vi "ARMS - LOCK.vi"(8 "error in (no error)":errorcluster, 9 "STATE":enum16{"LOCK", "UNLOCK"}(ring), 11 "SIDE":enum16{"LEFT", "RIGHT"}(ring)) -> (0 "error out":errorcluster, 3 "GET value":bool, 4 "previous GET\nvalue":bool)   [LabVIEW 2023]
uses:
  Global INIT.vi
  <vilib>/Rock Robotics/WPI/Solenoid/WPI_SolenoidValue.ctl
  <vilib>/Rock Robotics/WPI/Solenoid/WPI_SolenoidSetEnum.vi
  Global stack names.vi
  <vilib>/Rock Robotics/WPI/Solenoid/Deprecated/WPI_SolenoidGetBool.vi
  <vilib>/Rock Robotics/Network Tables/NT Write Boolean.vi
panel:
  out "stack name\nfor ARM LOCK":string
  out "INTENT":string
  out "Installed?":bool
  out "description":string
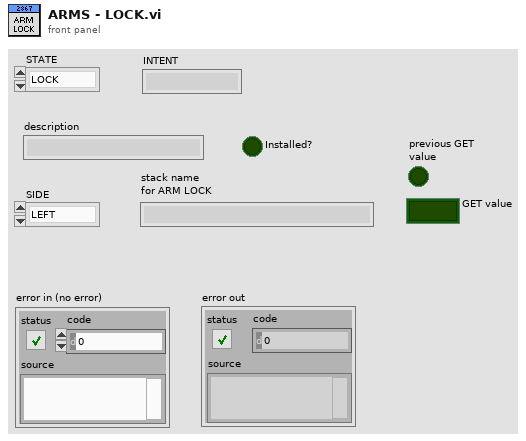
[diagram p1: front panel]
types:
  T1 = typedef "ctrl stack - ARMS.ctl" = cluster{"ARM LOCK":string, "ARM LIMIT EXTEND":string, "ARM LIMIT RETRACT ":string, "ARM EXTEND ":string, "ARM RETRACT":string}
  T2 = typedef "ctrl solenoid.ctl" = cluster{"description":string, "Installed?":bool, "refnum name":string, "coils":enum16{"Single", "Double"}, "forward channel":T3, "reverse channel":T3, "initial value":T4}
  T3 = typedef "WPI_SolenoidChannel.ctl" = enum8{"Solenoid 0", "Solenoid 1", "Solenoid 2", "Solenoid 3", "Solenoid 4", "Solenoid 5", "Solenoid 6", "Solenoid 7", "Solenoid 8", "Solenoid 9", "Solenoid 10", "Solenoid 11", "Solenoid 12", "Solenoid 13", "Solenoid 14", "Solenoid 15", "Invalid"}
  T4 = typedef "WPI_SolenoidValue.ctl" = enum16{"Off", "On", "Forward", "Reverse"}
  T5 = typedef "WPI_SolenoidDevRef.ctl" = cluster{"DevStatus":errorcluster, "Pneumatics Control Module":u8, "Forward Solenoid Channel":T3, "Reverse Solenoid Channel":T3}
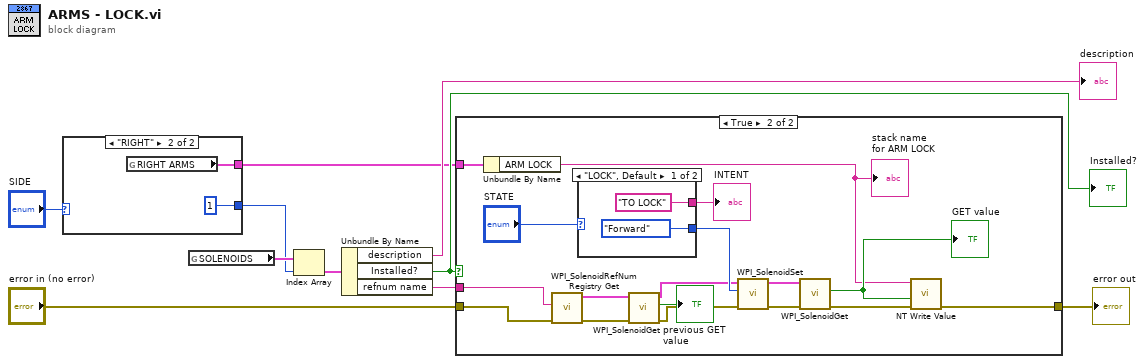
[diagram p0: block diagram]
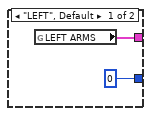
[diagram p2: hidden frame]
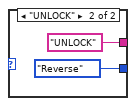
[diagram p4: hidden frame]
diagram:
  n1 = case shown="\"RIGHT\"" "SIDE" {
    tunnel: [0 1] -> w2
    tunnel: [w11 w13] -> w1
    frame "LEFT", Default {
      n2 = global read "Global stack names.vi" "LEFT ARMS"() -> (w11:T1)
    }
    frame "RIGHT" {
      n3 = global read "Global stack names.vi" "RIGHT ARMS"() -> (w13:T1)
    }
  }
  n4 = global read "Global INIT.vi" "SOLENOIDS"() -> (w10:T2[])
  n5 = Index Array(array=w10, index=w2) -> (element=w9:T2)
  n6 = Unbundle By Name(w9) -> ("description"=→"description":string, "Installed?"=w7:bool, "refnum name"=w6:string)
  "Installed?" <- w7
  n7 = case shown="True" w7 {
    tunnel: w6 -> [_ w31]
    tunnel: "error in (no error)" -> [_ w27]
    tunnel: [_ w20] -> w5
    tunnel: w1 -> [_ w23]
    frame False {
    }
    frame True {
      n8 = Unbundle By Name(w23) -> ("ARM LOCK"=w22:string)
      "stack name\nfor ARM LOCK" <- w22
      n9 = call <vilib>:"WPI_SolenoidRefNum Registry Get.vi"("error in (no error)"=w27, "refnum name"=w31) -> ("error out"=w17:errorcluster, "SolenoidDevRef"=w30:T5)  [unwired: 8 in]
      n10 = case shown="\"LOCK\", Default" "STATE" {
        tunnel: [WPI_SolenoidValue."Forward" ("Value") WPI_SolenoidValue."Reverse" ("Value")] -> w28
        tunnel: ["TO LOCK" "UNLOCK"] -> w19
        frame "LOCK", Default {
        }
        frame "UNLOCK" {
        }
      }
      "INTENT" <- w19
      n11 = call-poly <vilib>:"WPI_SolenoidGet.vi"("error in (no error)"=w17, "SolenoidDevRef"=w30) -> ("error out"=w16:errorcluster, "Value"=→"previous GET\nvalue":bool, "SolenoidDevRef"=w18:T5)  [unwired: 7 in]
      n12 = call-poly <vilib>:"WPI_SolenoidSet.vi"("error in (no error)"=w16, "Value"=w28, "SolenoidDevRef"=w18) -> ("error out"=w26:errorcluster, "SolenoidDevRef"=w25:T5)  [unwired: 7 in]
      n13 = call-poly <vilib>:"WPI_SolenoidGet.vi"("error in (no error)"=w26, "SolenoidDevRef"=w25) -> ("error out"=w21:errorcluster, "Value"=w24:bool)  [unwired: 7 in, 1 out]
      "GET value" <- w24
      n14 = call-poly <vilib>:"NT Write Value.vi"("error in"=w21, "value"=w24, "name"=w22) -> ("error out"=w20:errorcluster)  [unwired: 8 in]
    }
  }
  "error out" <- w5
